vi "Queue Nested.vi"(8 "Alias":string, 9 "Priority?":bool, 10 "Msg":refnum<class "Msg.lvclass">, 11 "jettl Event Actor in":refnum<class "jettl Event Actor.lvclass">) -> (3 "jettl Event Actor out":refnum<class "jettl Event Actor.lvclass">)   [LabVIEW 2021, in "jettl.lvlib" / "jettl Event Actor.lvclass"]
uses:
  jettl Event Actor.lvclass
  Actor/Msg/Msg.lvclass
  jettl Event Actor.lvclass/jettl Event Actor.ctl
  jettl.lvlib
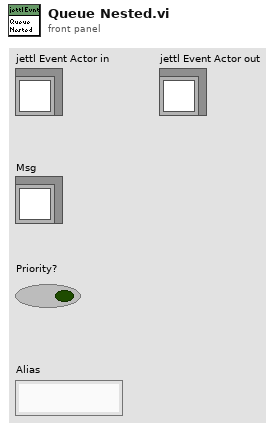
[diagram p1: front panel]
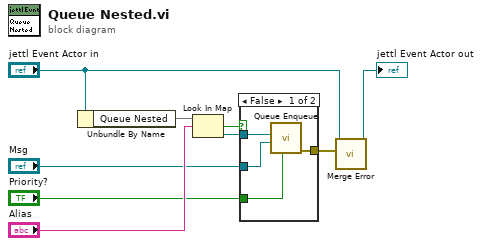
[diagram p0: block diagram]
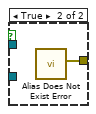
[diagram p2: hidden frame]
diagram:
  n1 = Unbundle By Name("jettl Event Actor in") -> ("Queue Nested"=w8:map{string, refnum<data-value>})
  n2 = Look In Map(map=w8, key="Alias") -> (key not found?=w7:bool, value=w9:refnum<data-value>)  [unwired: 1 in]
  n3 = case shown="False" w7 {
    tunnel: [w13 w14] -> w6
    tunnel: "Priority?" -> [w12 _]
    tunnel: "Msg" -> [w11 _]
    tunnel: w9 -> [w10 _]
    frame False {
      n4 = call "Queue Enqueue.vi"("Priority?"=w12, "Msg"=w11, "Queue"=w10) -> ("error out"=w13:errorcluster)  [unwired: 8 in]
    }
    frame True {
      n5 = call "Alias Does Not Exist Error.vi"() -> ("Error"=w14:errorcluster)  [unwired: 11 in]
    }
  }
  n6 = call-dynamic "Merge Error.vi"("Error"=w6, "Set Error in"="jettl Event Actor in") -> ("Set Error out"=→"jettl Event Actor out":refnum<class "jettl Event Actor.lvclass">)  [unwired: 9 in]
